vi "Query.vi"(8 "error in":errorcluster, 10 "Write in":string, 11 "6700C in":refnum<class "6700C.lvclass">) -> (0 "error out":errorcluster, 2 "Read out":string, 3 "6700C out":refnum<class "6700C.lvclass">)   [LabVIEW 2019, in "6700C.lvlib" / "6700C.lvclass"]
uses:
  Library/6700C.lvclass
  Library/6700C.lvclass/6700C.ctl
  <instrlib>/Agilent N6700 Series/Agilent N6700 Series.lvlib
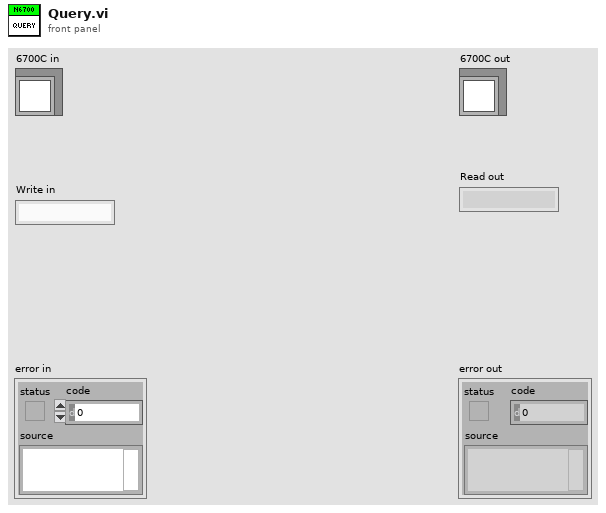
[diagram p1: front panel]
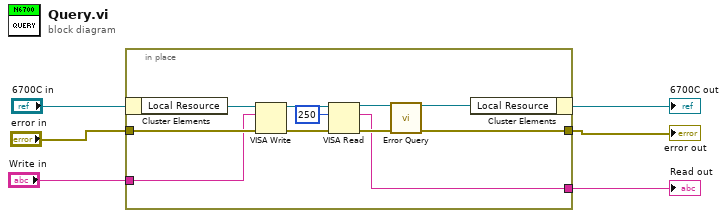
[diagram p0: block diagram]
diagram:
  n1 = in-place {
    in-place-border: "error in" -> [w16]
    in-place-border: "Write in" -> [w15]
    in-place-border: [w9] -> w2
    in-place-border: [w8] -> w1
    n2 = in-place-cluster #1("6700C in") -> ("Local Resource"=w17:refnum<visa-resource-name>)
    n3 = VISA Write(VISA resource name=w17, write buffer=w15, error in (no error)=w16) -> (VISA resource name out=w14:refnum<visa-resource-name>, error out=w13:errorcluster)  [unwired: 1 out]
    n4 = VISA Read(VISA resource name=w14, byte count=u32 250, error in (no error)=w13) -> (VISA resource name out=w11:refnum<visa-resource-name>, read buffer=w8:string, error out=w12:errorcluster)  [unwired: 1 out]
    n5 = call <instrlib>:"Error Query.vi"("VISA resource name"=w11, "error in (no error)"=w12) -> ("VISA resource name out"=w10:refnum<visa-resource-name>, "error out"=w9:errorcluster)  [unwired: 10 in, 2 out]
    n6 = in-place-cluster #1("Local Resource"=w10) -> (→"6700C out":refnum<class "6700C.lvclass">)
  }
  "error out" <- w2
  "Read out" <- w1
